vi "osc_test.vi"() -> ()   [LabVIEW 2016]
uses:
  xcontrol/Start Button.xctl
  <instrlib>/Tektronix TDS 200 1000 2000 Series/Public/Data/Read (Single Waveform).vi
  <instrlib>/Tektronix TDS 200 1000 2000 Series/Tektronix TDS 200 1000 2000 Series.lvlib
panel:
  out "Waveform Data":waveform(dbl)(graph)
  in  "Osiloskop Portu":refnum<visa-resource-name>="USB0::0x0699::0x0363::C102985::INSTR"
  in  "Start Button":dbl(xcontrol)
  in  "Reset Dafault":bool
  in  "cmdOrjin":bool
  in  "cmdStop":bool
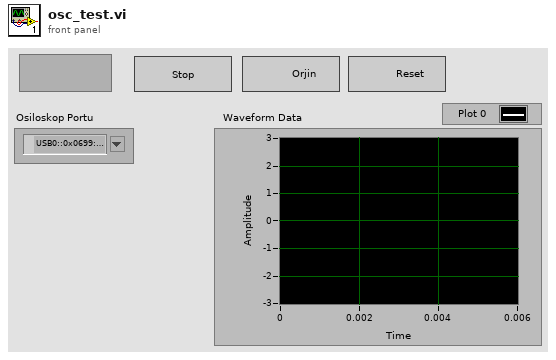
[diagram p1: front panel]
types:
  T1 = cluster{"Baud Rate":u32, "Parity":u16, "Stop Bits":u16, "Flow Control":u16}
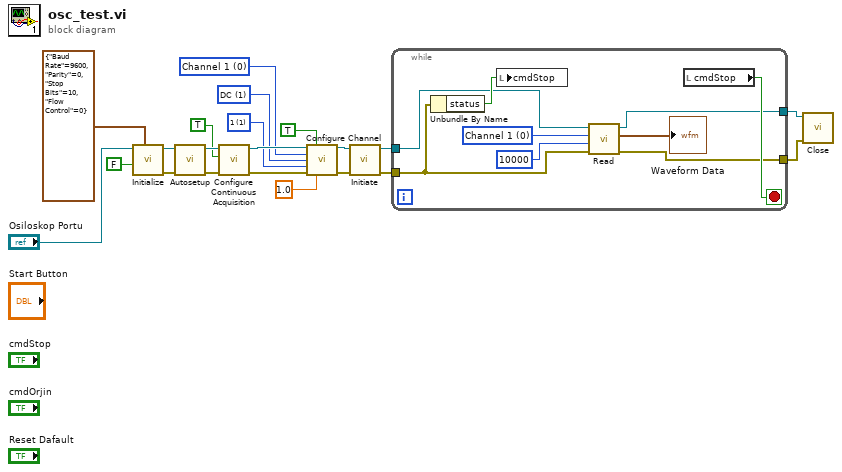
[diagram p0: block diagram]
diagram:
  w5 = 1 items=["AC", "DC", "Ground"] ("Vertical Coupling (1: DC)")
  w6 = 0 items=["Channel 1", "Channel 2", "Channel 3", "Channel 4", "Math", "Reference A", "Reference B", "Reference C", "Reference D"] ("Channel (0: Channel 1)")
  w8 = 1 items=["1"=1, "10"=10, "20"=20, "50"=50, "100"=100, "500"=500, "1000"=1000] ("Probe Attenuation (10: 10X)")
  n1 = call <instrlib>:"Initialize.vi"("Serial Configuration"=T1 {"Baud Rate"=9600, "Parity"=0, "Stop Bits"=10, "Flow Control"=0} ("Osiloskop Config"), "Reset? (T: Yes)"=FALSE, "VISA resource name"="Osiloskop Portu") -> ("error out"=w17:errorcluster, "VISA resource name out"=w18:refnum<visa-resource-name>)  [unwired: 2 in, 5 out]
  n2 = call <instrlib>:"Autosetup.vi"("error in (no error)"=w17, "VISA resource name"=w18) -> ("error out"=w19:errorcluster, "VISA resource name out"=w20:refnum<visa-resource-name>)  [unwired: 8 out]
  n3 = call <instrlib>:"Configure Continuous Acquisition.vi"("error in (no error)"=w19, "Enable Continuous Acquisition Mode (True)"=TRUE, "VISA resource name"=w20) -> ("error out"=w9:errorcluster, "VISA resource name out"=w12:refnum<visa-resource-name>)  [unwired: 7 out]
  n4 = call <instrlib>:"Configure Channel.vi"("VISA resource name"=w12, "Enable Channel (True)"=TRUE, "Channel (0: Channel 1)"=w6, "Vertical Coupling (1: DC)"=w5, "Probe Attenuation (10: 10X)"=w8, "error in (no error)"=w9, "Vertical Range (10.0 V/div)"=1.0) -> ("VISA resource name out"=w11:refnum<visa-resource-name>, "error out"=w10:errorcluster)  [unwired: 7 in]
  n5 = call <instrlib>:"Initiate.vi"("error in (no error)"=w10, "VISA resource name"=w11) -> ("error out"=w13:errorcluster, "VISA resource name out"=w14:refnum<visa-resource-name>)  [unwired: 8 out]
  n6 = while {
    tunnel: w14 -> [w25]
    tunnel: w13 -> [w24]
    tunnel: [w23] -> w2
    tunnel: [w22] -> w1
    stop <- w30 stop-if-true
    w27 = u16 0 items=["Channel 1", "Channel 2", "Channel 3", "Channel 4", "Math", "Reference A", "Reference B", "Reference C", "Reference D"] ("Channel B (1: Channel 2)")
    n7 = Unbundle By Name(w24) -> ("status"=w29:bool)
    n8 = local write "cmdStop"(w29) -> ()
    n9 = call-poly <instrlib>:"Read.vi"("error in (no error)"=w24, "Timeout (10000 ms)"=u32 10000 ("Timeout (10000 ms) 2"), "Source (0: Channel 1)"=w27, "VISA resource name"=w25) -> ("error out"=w22:errorcluster, "Waveform Data"=→"Waveform Data":waveform(dbl), "VISA resource name out"=w23:refnum<visa-resource-name>)  [unwired: 5 out]
    n10 = local read "cmdStop"() -> (w30:bool)
  }
  n11 = call <instrlib>:"Close.vi"("error in (no error)"=w1, "VISA resource name"=w2) -> ()  [unwired: 9 in, 1 out]
